vi "test_Format Instrument String Response_Single Channel Data Type.vi"(8 "error in (no error)":errorcluster, 11 "TestCase in":refnum<class "Instrument Addon Unit Tests.lvclass">) -> (0 "error out":errorcluster, 3 "TestCase out":refnum<class "Instrument Addon Unit Tests.lvclass">)   [LabVIEW 2019, in "Instrument Addon Unit Tests.lvclass"]
uses:
  Instrument Addon Unit Tests.lvclass
  Addon/Addon Shared/Types/Response RT Configuration Cluster.ctl
  Addon/Addon Shared/Types/Response Parameters.ctl
  Addon/Addon Shared/Types/Linked Channel Cluster.ctl
  Addon/Addon Shared/Types/Response Wait Type.ctl
  <vilib>/addons/_JKI Toolkits/VI Tester/TestCase.llb/TestCase.lvclass
  Addon/Addon Engine/Instrument Addon Engine.lvlib
  Addon/Addon Shared/Instrument Addon Shared.lvlib
  C:/Program Files (x86)/National Instruments/LabVIEW 2019/vi.lib/addons/_JKI Toolkits/VI Tester/TestCase.llb/TestCase.lvclass
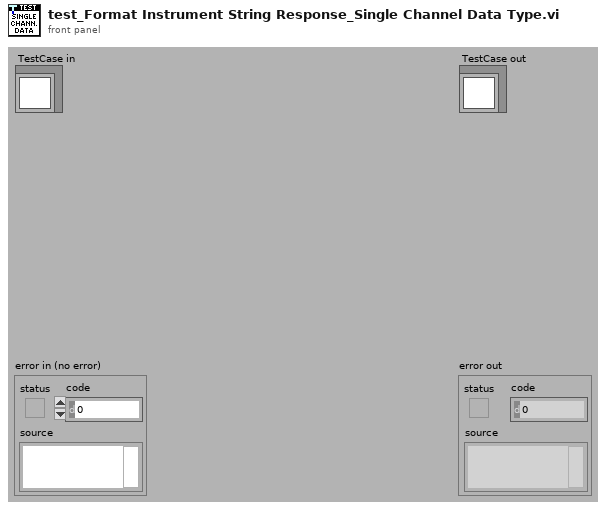
[diagram p1: front panel]
types:
  T1 = typedef "Instrument Addon Shared.lvlib/Response RT Configuration Cluster.ctl" = cluster{"Reponse Parameters":T2, "Use?":bool}
  T2 = typedef "Instrument Addon Shared.lvlib/Response Parameters.ctl" = cluster{"Response":string, "Linked Channels":T3[], "Type Value":dbl, "Wait Type":T4, "Use Channel":bool, "Channel Path":string}
  T3 = typedef "Instrument Addon Shared.lvlib/Linked Channel Cluster.ctl" = cluster{"Variable Name":string, "GUID":string}
  T4 = typedef "Instrument Addon Shared.lvlib/Response Wait Type.ctl" = enum16{"Byte Count", "Wait sec"}
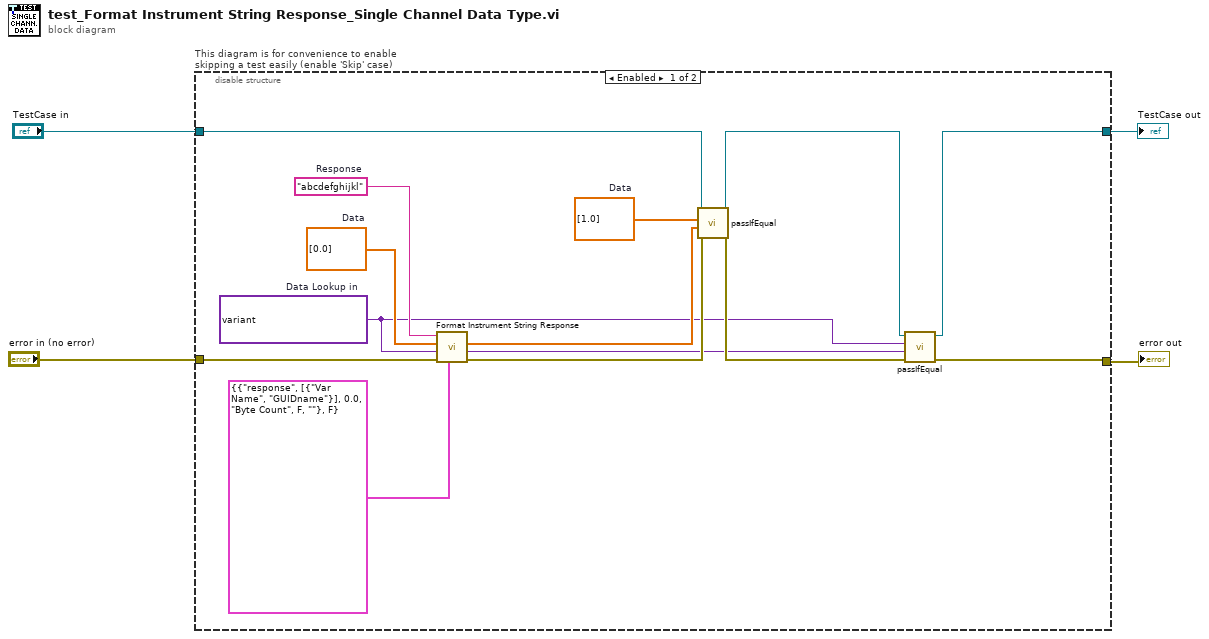
[diagram p0: block diagram]
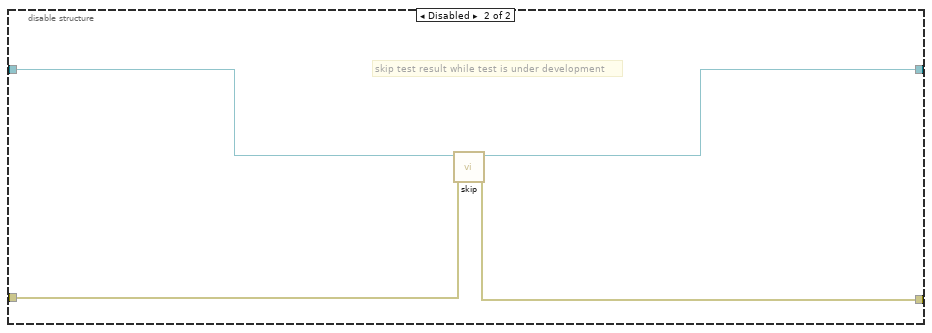
[diagram p2: hidden frame]
diagram:
  n1 = disable-structure "This diagram is for convenience to enable skipping a test easily (enable 'Skip' case)" shown="Enabled" {
    disable-tunnel: "TestCase in" -> [w18 w22]
    disable-tunnel: [w14 w20] -> w1
    disable-tunnel: [w16 w21] -> w3
    disable-tunnel: "error in (no error)" -> [w12 w19]
    frame Enabled {
      w6 = dbl[] [1.0]  # Data
      w7 = variant("GUIDname"=variant(cluster{"Data Parameters":cluster{"Data Type":enum16{"Single Channel", "Array"}, "Channel Type":enum16{"Format", "Comparison", "Type Cast", "Enumerated List"}, "Format String":string, "Expected String":string, "Type":enum16{"DBL", "SGL", "U64", "U32", "U16", "U8", "I64", "I32", "I16", "I8"}, "List":string[], "Delimiter":string, "Endian":enum16{"Native", "Little", "Big"}}, "Data Index":i32, "Data Length":i32} {"Data Parameters"={"Data Type"=enum."Single Channel", "Channel Type"=enum."Comparison", "Format String"="%s", "Expected String"="bcd", "Type"=enum."SGL", "List"=[], "Delimiter"="", "Endian"=enum."Native"}, "Data Index"=0, "Data Length"=0}))  # Data Lookup in
      w8 = dbl[] [0.0]  # Data
      w9 = "abcdefghijkl"  # Response
      n2 = call "Format Instrument String Response.vi"("Response Parameters"=T1 {"Reponse Parameters"={"Response"="response", "Linked Channels"=[{"Variable Name"="Var Name", "GUID"="GUIDname"}], "Type Value"=0.0, "Wait Type"=enum."Byte Count", "Use Channel"=FALSE, "Channel Path"=""}, "Use?"=FALSE}, "error in (no error)"=w12, "Data Lookup in"=w7, "Data"=w8, "Response"=w9) -> ("error out"=w13:errorcluster, "Data Lookup out"=w11:variant, "Data out"=w10:dbl[])  [unwired: 4 in]
      n3 = call-dynamic "passIfEqual.vi"("error in (no error)"=w13, "y"=w10, "x"=w6, "TestCase in"=w18) -> ("error out"=w17:errorcluster, "TestCase out"=w15:refnum<class "Instrument Addon Unit Tests.lvclass">)  [unwired: 6 in]
      n4 = call-dynamic "passIfEqual.vi"("error in (no error)"=w17, "y"=w11, "x"=w7, "TestCase in"=w15) -> ("error out"=w16:errorcluster, "TestCase out"=w14:refnum<class "Instrument Addon Unit Tests.lvclass">)  [unwired: 6 in]
    }
    frame Disabled {
      # "skip test result while test is under development"
      n5 = call <vilib>:"skip.vi"("error in (no error)"=w19, "TestCase in"=w22) -> ("error out"=w21:errorcluster, "TestCase out"=w20:refnum<class "Instrument Addon Unit Tests.lvclass">)  [unwired: 8 in]
    }
  }
  "error out" <- w3
  "TestCase out" <- w1
